vi "Error 6000 -- Unexpected Door Interlock Value.vi"(8 "error in (no error)":errorcluster, 9 "Interlock Value":bool, 10 "Interlock Name":T1, 11 "Door Controller":refnum<class "Door Controller.lvclass">) -> (0 "error out":errorcluster)   [LabVIEW 2020, in "Application.lvlib"]
uses:
  Application.lvlib
  Door Controller/Door Controller/Door Controller.lvclass
  Interlock Names.ctl
  <vilib>/Utility/error.llb/Error Cluster From Error Code.vi
  <vilib>/ErrorRing/Error Ring.xnode
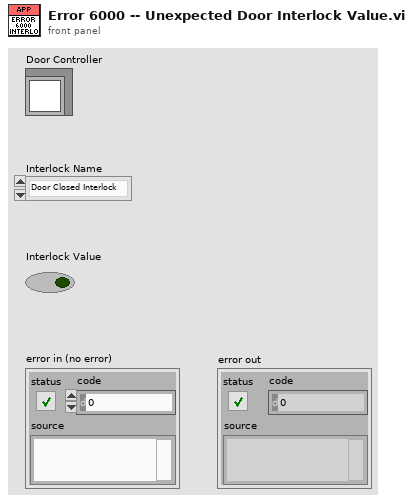
[diagram p1: front panel]
types:
  T1 = typedef "Application.lvlib/Interlock Names.ctl" = enum16{"Door Closed Interlock", "Door Open Interlock"}
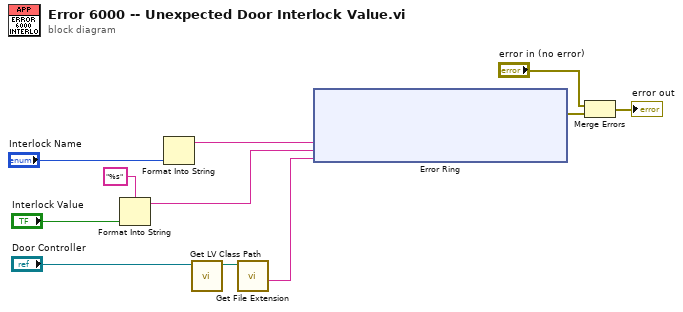
[diagram p0: block diagram]
diagram:
  n1 = Format Into String(format string="%s", "Interlock Value") -> (resulting string=w8:string)  [unwired: 2 in, 1 out]
  n2 = Format Into String("Interlock Name") -> (resulting string=w3:string)  [unwired: 3 in, 1 out]
  n3 = call <vilib>:"Get LV Class Path.vi"("object"="Door Controller") -> ("class path"=w7:path)  [unwired: 9 in, 1 out]
  n4 = call <vilib>:"Get File Extension.vi"("file"=w7) -> ("filename without extension"=w6:string)  [unwired: 6 in, 4 out]
  n5 = xnode "Error Ring"("parameter 0"=w3, "parameter 1"=w8, "parameter 2"=w6) -> ("error out"=w11:errorcluster)
  n6 = Merge Errors("error in (no error)", w11) -> (→"error out":errorcluster)
